vi "CSM-LogViewer.vi"() -> ()   [LabVIEW 2020]
uses:
  Typedef/Def - CSMLog Line - Cluster.ctl
  Typedef/Def - CSMLog Line - File Info - Cluster.ctl
  <userlib>/_NEVSTOP/Communicable State Machine(CSM)/_Support/Priority Queue/Priority Queue.lvclass/Priority Queue.ctl
  5abc820e-fff5-455f-84ac-6161549f095a.vi
  d19c4e55-5bdc-402e-9f7e-e2ad1133e7d6.vi
  <userlib>/_NEVSTOP/Communicable State Machine(CSM)/_Support/Process/CSMP-Async Call.vi
  <userlib>/_NEVSTOP/Communicable State Machine(CSM)/_Support/GlobalEvent/GEvt-Generate Status Log.vi
  <userlib>/_NEVSTOP/Communicable State Machine(CSM)/_Support/Process/CSMP-Broadcast.vi
  <userlib>/_NEVSTOP/Communicable State Machine(CSM)/_Support/GlobalEvent/GEvt-Generate Interrupt Log.vi
  <userlib>/_NEVSTOP/Communicable State Machine(CSM)/_Support/GlobalEvent/GEvt-Generate Register Log.vi
  <userlib>/_NEVSTOP/Communicable State Machine(CSM)/_Support/Process/CSMP-Register Status.vi
  <userlib>/_NEVSTOP/Communicable State Machine(CSM)/_Support/GlobalEvent/GEvt-Generate Unregister Log.vi
  <userlib>/_NEVSTOP/Communicable State Machine(CSM)/_Support/Process/CSMP-Unregister Status.vi
  <userlib>/_NEVSTOP/Communicable State Machine(CSM)/_Support/Process/CSMP-Sync Call.vi
  <userlib>/_NEVSTOP/Communicable State Machine(CSM)/_Support/CSMQ/_CSMObj-Unlock.vi
  <userlib>/_NEVSTOP/Communicable State Machine(CSM)/_Support/Process/CSMP-PostPostMsg.vi
  <userlib>/_NEVSTOP/Communicable State Machine(CSM)/_Support/Process/CSMP-PostSendMsg.vi
  <userlib>/_NEVSTOP/Communicable State Machine(CSM)/_Support/CSMQ/_CSMObj-Lock State.vi
  <userlib>/_NEVSTOP/Communicable State Machine(CSM)/_Support/Common/Splite Reason String Part.vi
  <userlib>/_NEVSTOP/Communicable State Machine(CSM)/_Support/Common/Trim Single line Text.vi
  <userlib>/_NEVSTOP/Communicable State Machine(CSM)/_Support/CSMQ/_CSMOFGV Release.vi
  <userlib>/_NEVSTOP/Communicable State Machine(CSM)/_Support/Common/Remove Comments from Line.vi
  <userlib>/_NEVSTOP/Communicable State Machine(CSM)/_Support/Common/Splite Single-line Message.vi
  <userlib>/_NEVSTOP/Communicable State Machine(CSM)/_Support/Common/Parse Next Single-line State.vi
  <userlib>/_NEVSTOP/Communicable State Machine(CSM)/_Support/CSMQ/_CSMOFGV Dequeue.vi
  <userlib>/_NEVSTOP/Communicable State Machine(CSM)/_Support/CSMQ/_CSMObj-Log Error if in a Remote Session.vi
  <userlib>/_NEVSTOP/Communicable State Machine(CSM)/_Support/GlobalEvent/GEvt-Generate State Change Log.vi
  <userlib>/_NEVSTOP/Communicable State Machine(CSM)/_Support/GlobalEvent/GEvt-Generate Remaining States Log.vi
  <userlib>/_NEVSTOP/Communicable State Machine(CSM)/_Support/GlobalEvent/GEvt-Generate Module Destroyed Log.vi
  <userlib>/_NEVSTOP/Communicable State Machine(CSM)/_Support/GlobalEvent/GEvt-Generate Complete Log.vi
  <userlib>/_NEVSTOP/Communicable State Machine(CSM)/_Support/GlobalEvent/GEvt-Generate Module Created Log.vi
  <userlib>/_NEVSTOP/Communicable State Machine(CSM)/_Support/Common/Format Timestamp.vi
  <userlib>/_NEVSTOP/Communicable State Machine(CSM)/AdvanceAPI/CSM - Revert Arguments-Safe String.vi
  <userlib>/_NEVSTOP/Communicable State Machine(CSM)/AdvanceAPI/CSM - Make String Arguments Safe.vi
  <userlib>/_NEVSTOP/Communicable State Machine(CSM)/AdvanceAPI/CSM - Break Down Multiple States String.vi
  <userlib>/_NEVSTOP/Communicable State Machine(CSM)/AdvanceAPI/CSM - Compact Multiple States.vi
  <userlib>/_NEVSTOP/Communicable State Machine(CSM)/_Support/CSMQ/_Obtain CSM Data Queue.vi
  <userlib>/_NEVSTOP/Communicable State Machine(CSM)/_Support/Priority Queue/Release Priority Queue.vi
  d19c4e55-5bdc-402e-9f7e-e2ad1133e7d6.vi/eb2405bd-5b2e-436b-9bb3-692ecf4a9268.vi
  d19c4e55-5bdc-402e-9f7e-e2ad1133e7d6.vi/c8ad12e3-5e6d-40e1-92e0-1426ef45ec41.vi
  d19c4e55-5bdc-402e-9f7e-e2ad1133e7d6.vi/effcbc1a-e97c-42d4-b61f-d821de102707.vi
  <userlib>/_NEVSTOP/Communicable State Machine(CSM)/_Support/CSMQ/_CSMObj-Message Check.vi
  <userlib>/_NEVSTOP/Communicable State Machine(CSM)/_Support/CSMQ/_CSMObj-Enqueue Cross-Module Message.vi
  <userlib>/_NEVSTOP/Communicable State Machine(CSM)/_Support/CSMQ/_CSMOFGV Get.vi
  <userlib>/_NEVSTOP/Communicable State Machine(CSM)/_Support/FGV-BroadcastRegistry/Cache-Broadcast Registry Search Result.vi
  <userlib>/_NEVSTOP/Communicable State Machine(CSM)/AdvanceAPI/CSM - Register Status Change.vi
  <userlib>/_NEVSTOP/Communicable State Machine(CSM)/AdvanceAPI/CSM - Unregister Status Change.vi
  <userlib>/_NEVSTOP/Communicable State Machine(CSM)/_Support/Common/Hex Str to U8 Data.vi
  <userlib>/_NEVSTOP/Communicable State Machine(CSM)/_Support/Common/Concatenate State with Arguments.vi
  <userlib>/_NEVSTOP/Communicable State Machine(CSM)/_Support/Common/U8 Data to Hex Str.vi
  <userlib>/_NEVSTOP/Communicable State Machine(CSM)/_Support/Priority Queue/Dequeue Element.vi
  <userlib>/_NEVSTOP/Communicable State Machine(CSM)/AdvanceAPI/CSM - Keywords.vi
  <userlib>/_NEVSTOP/Communicable State Machine(CSM)/_Support/Priority Queue/Obtain Priority Queue.vi
  <userlib>/_NEVSTOP/Communicable State Machine(CSM)/_Support/Priority Queue/Enqueue Element.vi
  <userlib>/_NEVSTOP/Communicable State Machine(CSM)/_Support/GlobalEvent/FGV-GlobalEventRef.vi
  <userlib>/_NEVSTOP/Communicable State Machine(CSM)/_Support/CSMQ/_CSMOFGV Obtain.vi
  <userlib>/_NEVSTOP/Communicable State Machine(CSM)/_Support/CSMQ/_CSMOFGV.vi
  <userlib>/_NEVSTOP/Communicable State Machine(CSM)/_Support/Error/CSM Not Allowed Message.vi
  <userlib>/_NEVSTOP/Communicable State Machine(CSM)/_Support/GlobalEvent/FGV-StatusChangeEventRef.vi
  <userlib>/_NEVSTOP/Communicable State Machine(CSM)/_Support/FGV-BroadcastRegistry/global-CSMQ FGV Change Flag.vi
  <userlib>/_NEVSTOP/Communicable State Machine(CSM)/_Support/FGV-BroadcastRegistry/global-Broadcast Cache Change Flag.vi
  <userlib>/_NEVSTOP/Communicable State Machine(CSM)/_Support/BroadcastRegistry/HelperVI/Broadcast Item Key.vi
  <userlib>/_NEVSTOP/Communicable State Machine(CSM)/_Support/FGV-BroadcastRegistry/FGV-BroadcastRegistry.vi
  <userlib>/_NEVSTOP/Communicable State Machine(CSM)/_Support/Message/Parse Register Message.vi
  <userlib>/_NEVSTOP/Communicable State Machine(CSM)/_Support/Message/Parse Unregister Message.vi
  <userlib>/_NEVSTOP/Communicable State Machine(CSM)/addons/API-String-Arugments-Support/_Support/Data To API String Arguments.vi
  <userlib>/_NEVSTOP/Communicable State Machine(CSM)/AdvanceAPI/CSM - Replace Substitution Marks in Messages.vi
  <userlib>/_NEVSTOP/Communicable State Machine(CSM)/_Support/Priority Queue/Priority Queue.lvclass
  <userlib>/_NEVSTOP/Communicable State Machine(CSM)/Communicable State Machine.lvlib
  71ee8597-0d9a-41c2-b129-d09668d4d4ef.vi
  <userlib>/_NEVSTOP/Communicable State Machine(CSM)/addons/API-String-Arugments-Support/API String Arguments Support.lvlib
  <userlib>/_NEVSTOP/Communicable State Machine(CSM)/addons/MassData-Parameter/CSM MassData Parameter Support.lvlib
panel:
  in  "Synchronize":bool
  in  "File Open":bool
  out "State History":string
  in  "Tree":string(tree)
  out "Variant":variant
  out "data":string
  out "offset (in bytes) (0)":i64 format="%.3p"
  out "size (in bytes)":i64 format="%.3p"
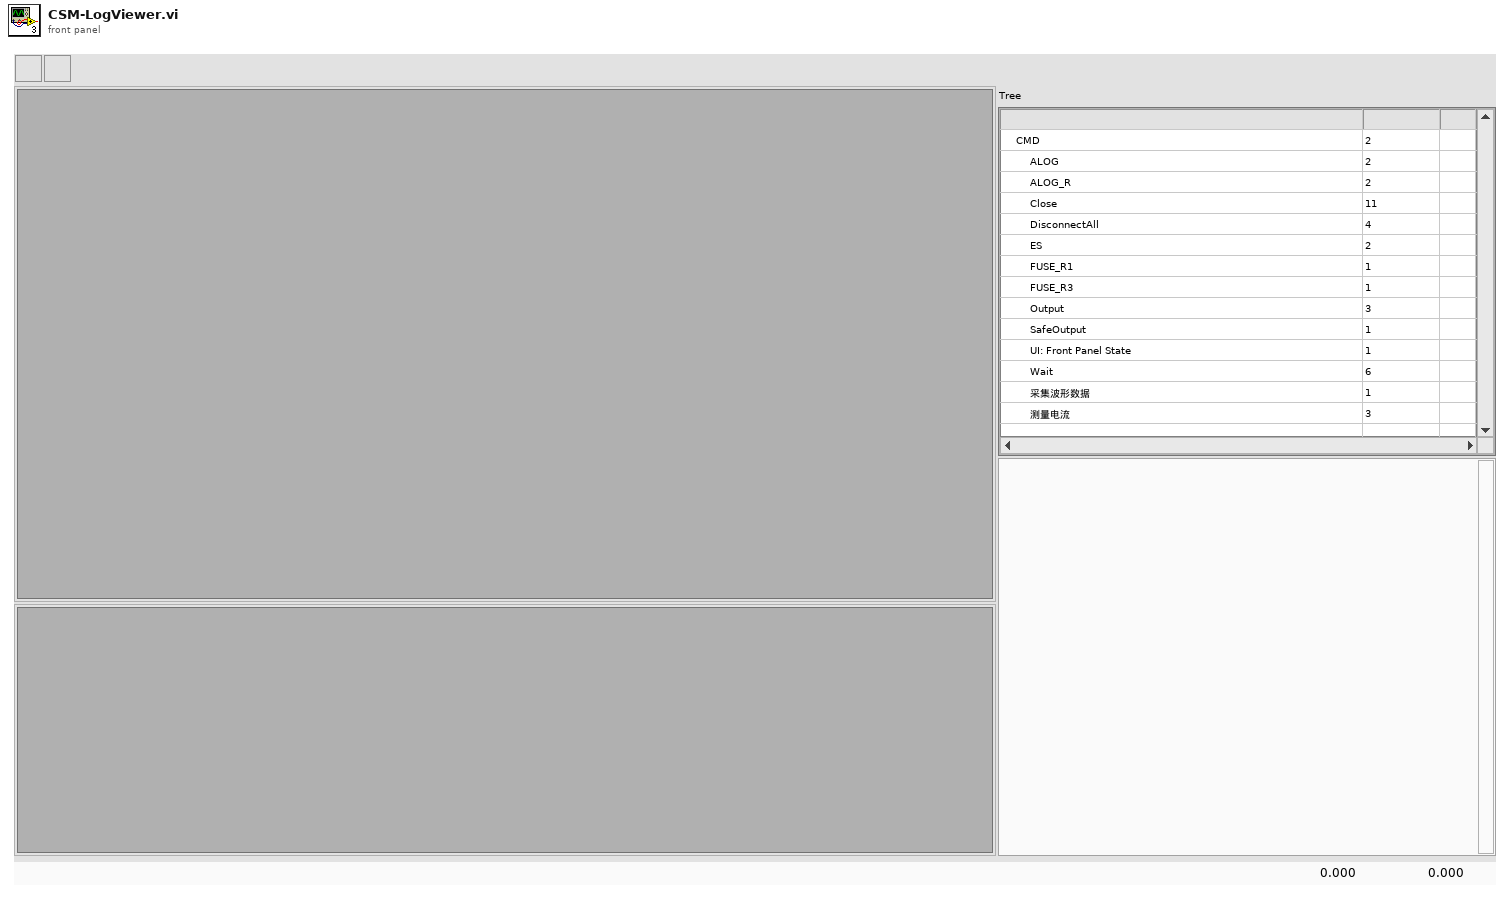
[diagram p1: front panel]
types:
  T1 = typedef "Def - CSMLog Line - Cluster.ctl" = cluster{"Content":string, "FileInfo":T2}
  T2 = typedef "Def - CSMLog Line - File Info - Cluster.ctl" = cluster{"Start":i32, "Length":i32}
  T3 = enum32{"Invalid", "Standard", "Closed", "Hidden", "Minimized", "Maximized"}
  T4 = enum32{"invalid app kind", "Development System", "Run Time System", "Student Edition", "Embedded LabVIEW", "Evaluation", "Custom"}
  T5 = typedef "Communicable State Machine.lvlib/_CSM_Response Source Message.ctl" = cluster{"‘State":string, "’Arguments":string, "’Error":errorcluster}
  T6 = cluster{"Core":cluster{"Current VI Reference":refnum<vi>, "Close Panel on Exit?":bool}, "Your Boolean data":bool, "Your string data":string}
  T7 = cluster{"Current VI Reference":refnum<vi>, "Close Panel on Exit?":bool}
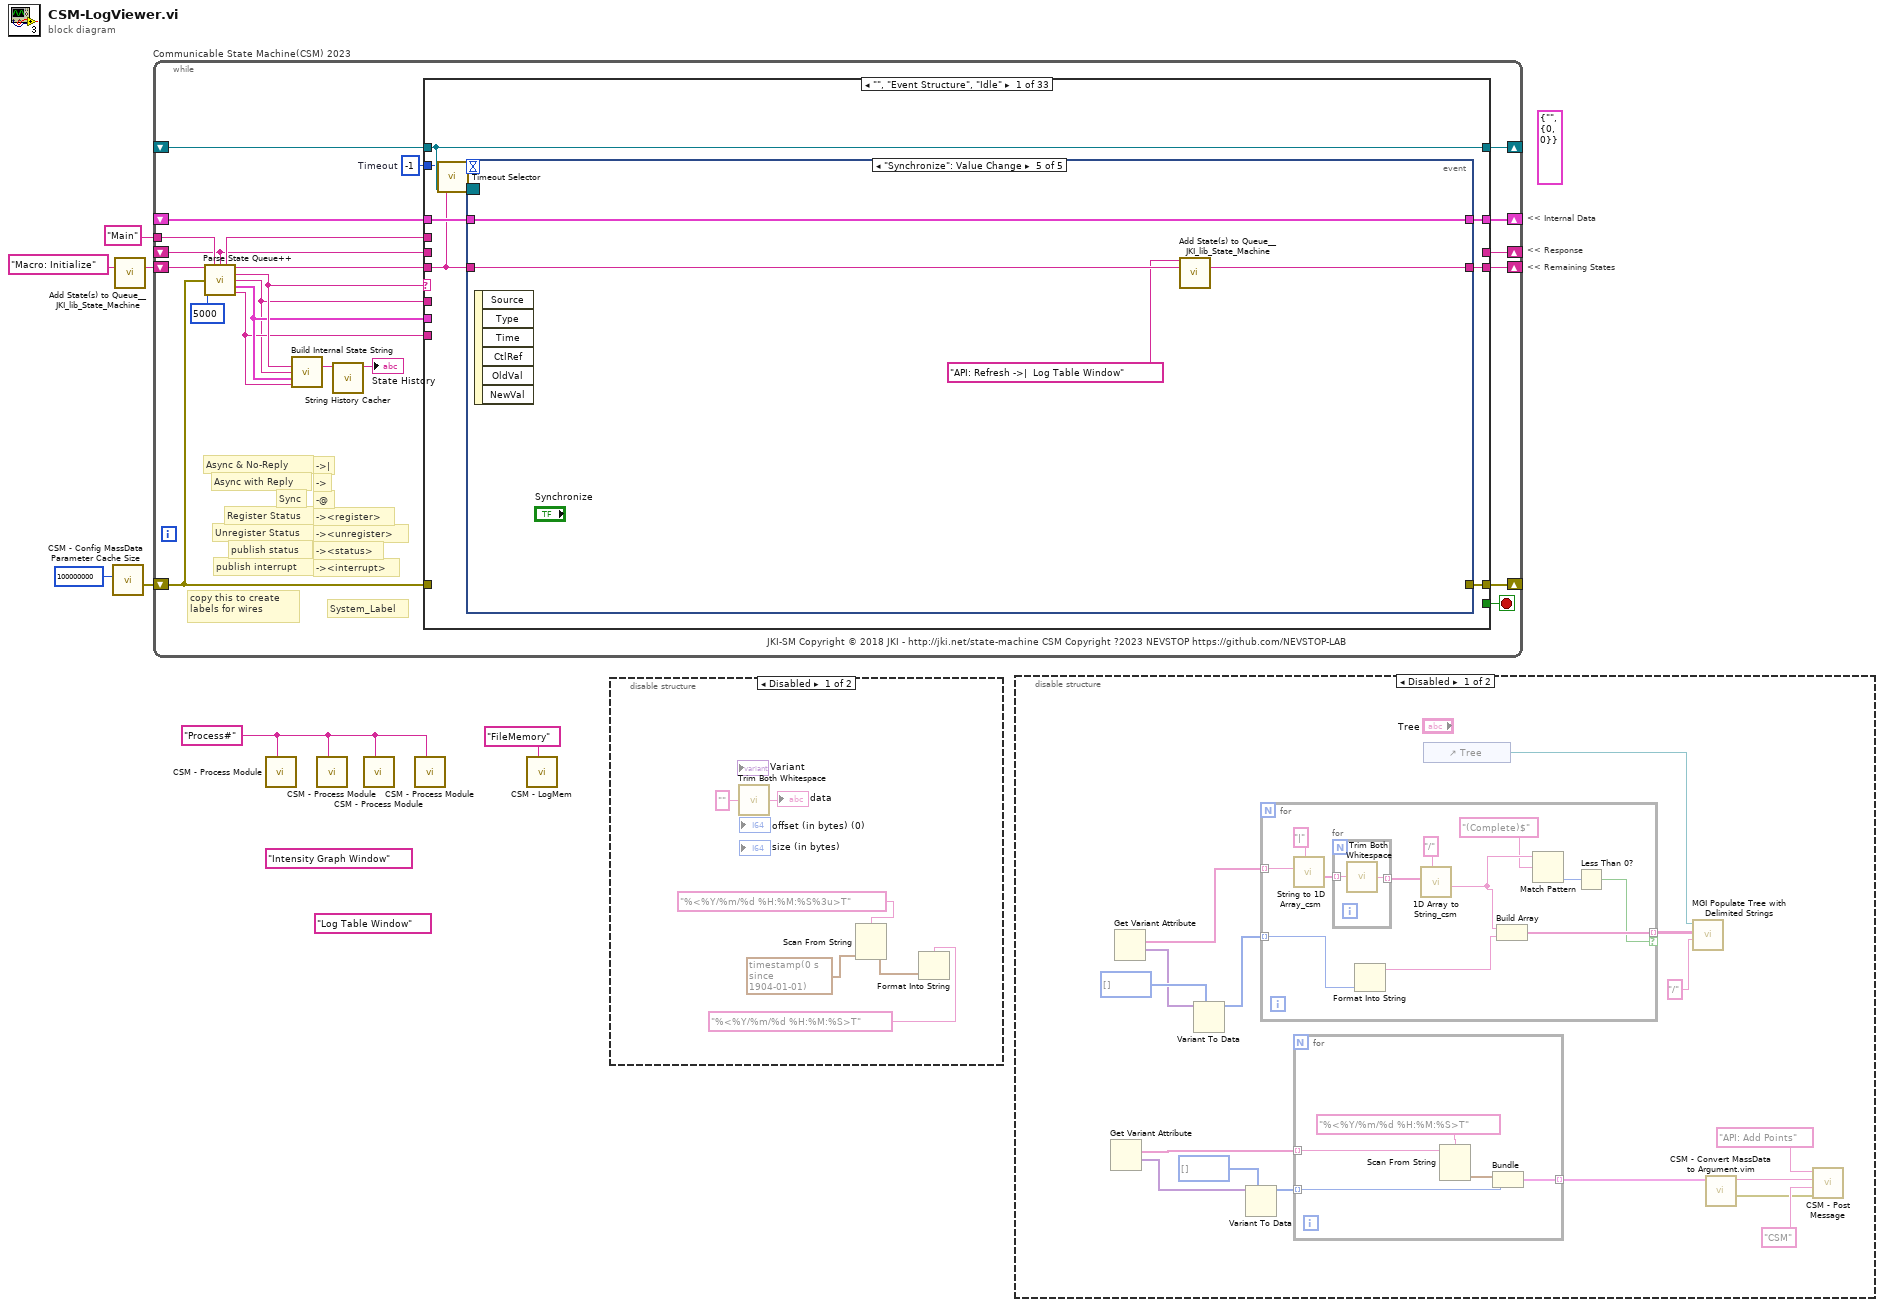
[diagram p0: block diagram]
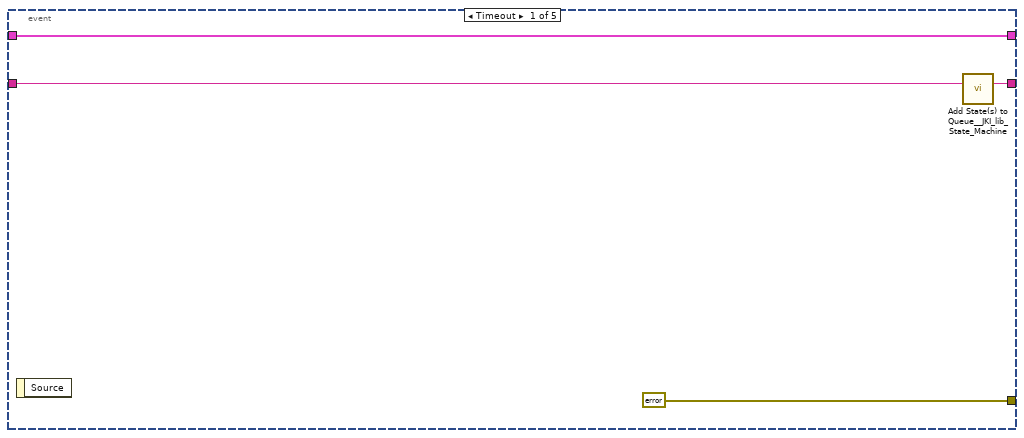
[diagram p4: hidden frame]
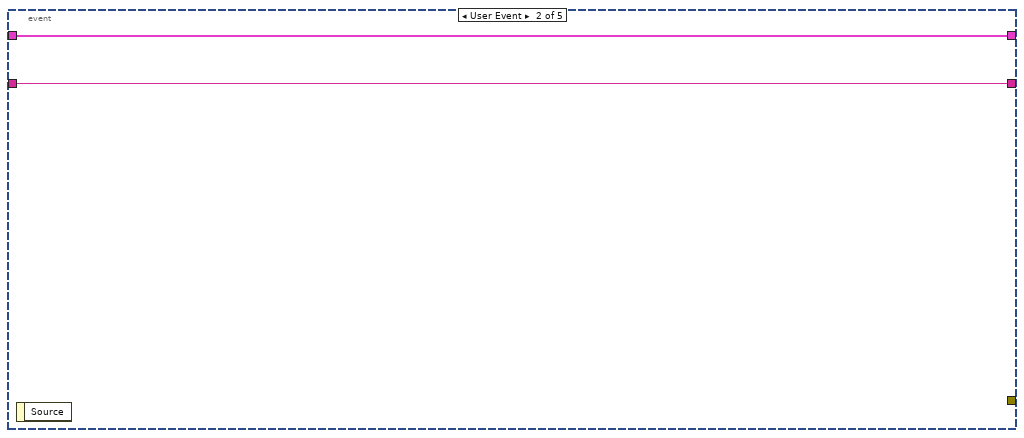
[diagram p5: hidden frame]
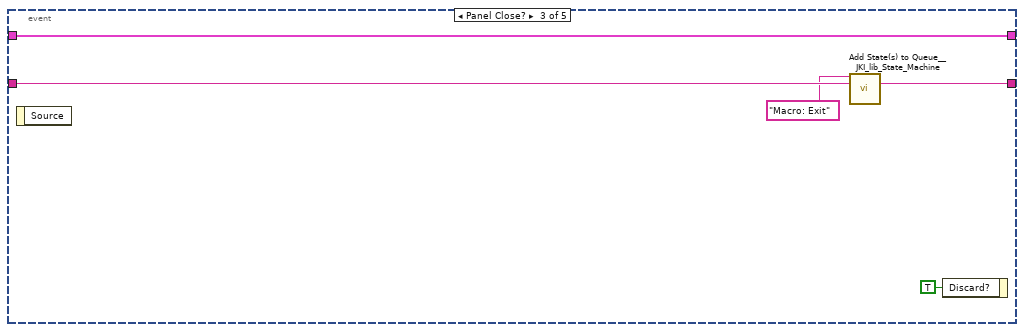
[diagram p6: hidden frame]
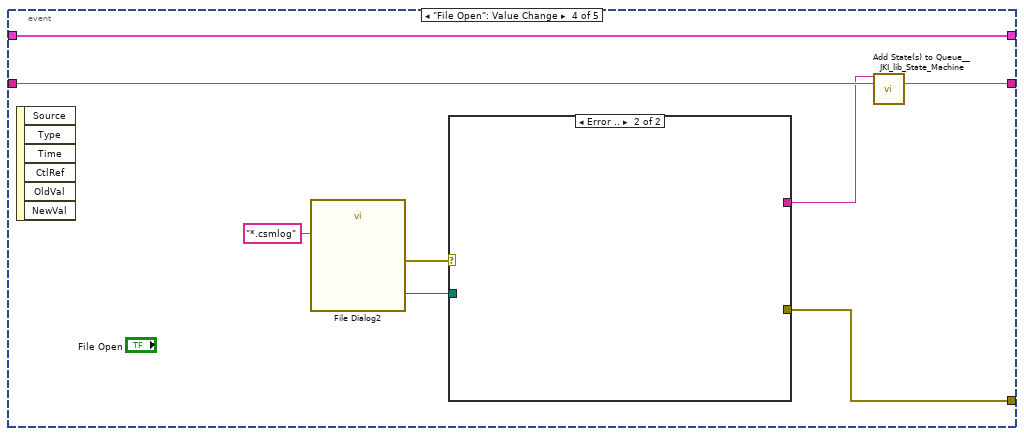
[diagram p7: hidden frame]
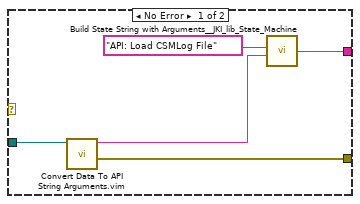
[diagram p8: hidden frame]
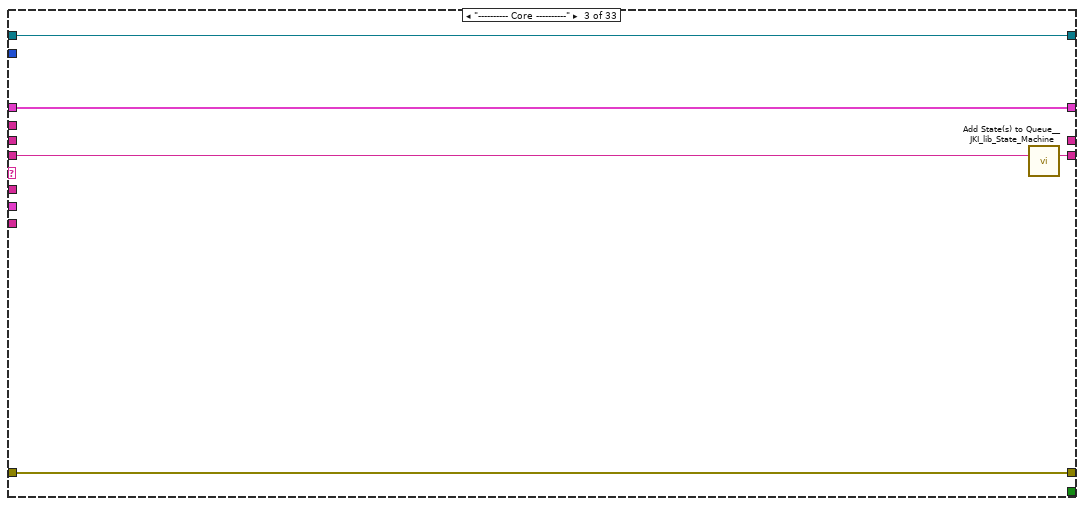
[diagram p10: hidden frame]
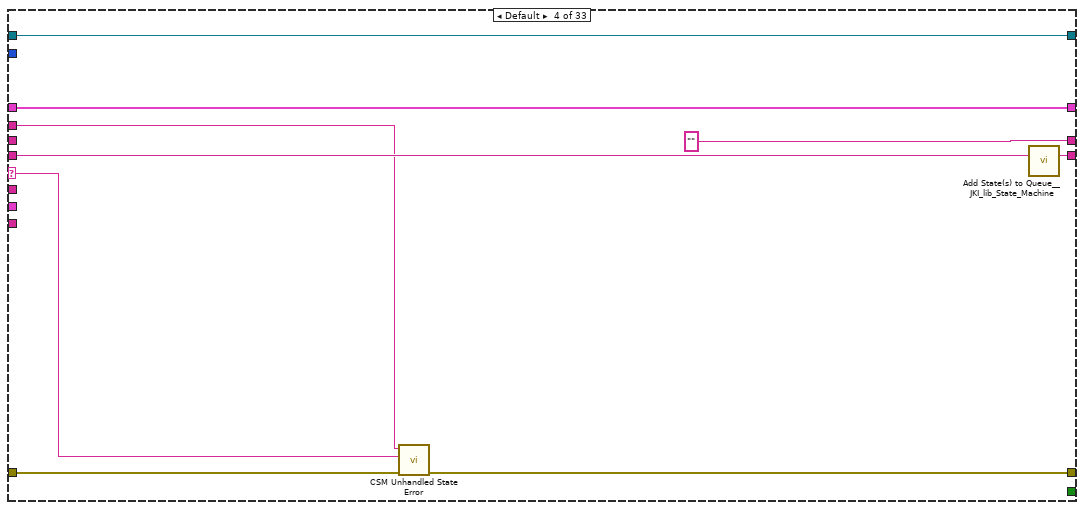
[diagram p11: hidden frame]
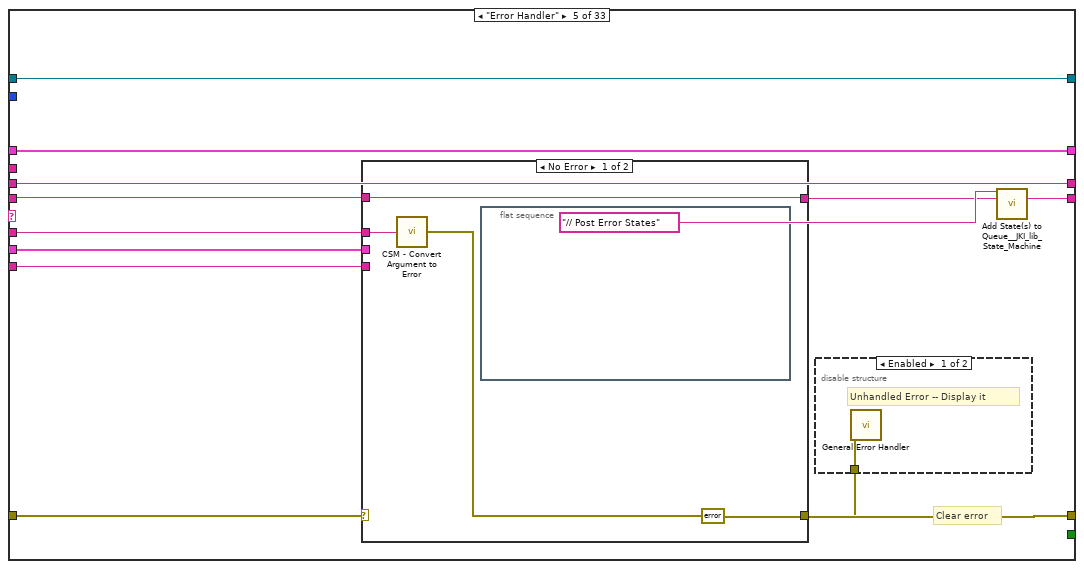
[diagram p12: hidden frame]
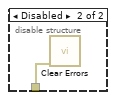
[diagram p13: hidden frame]
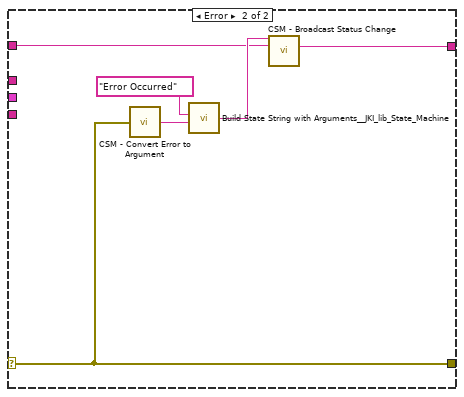
[diagram p14: hidden frame]
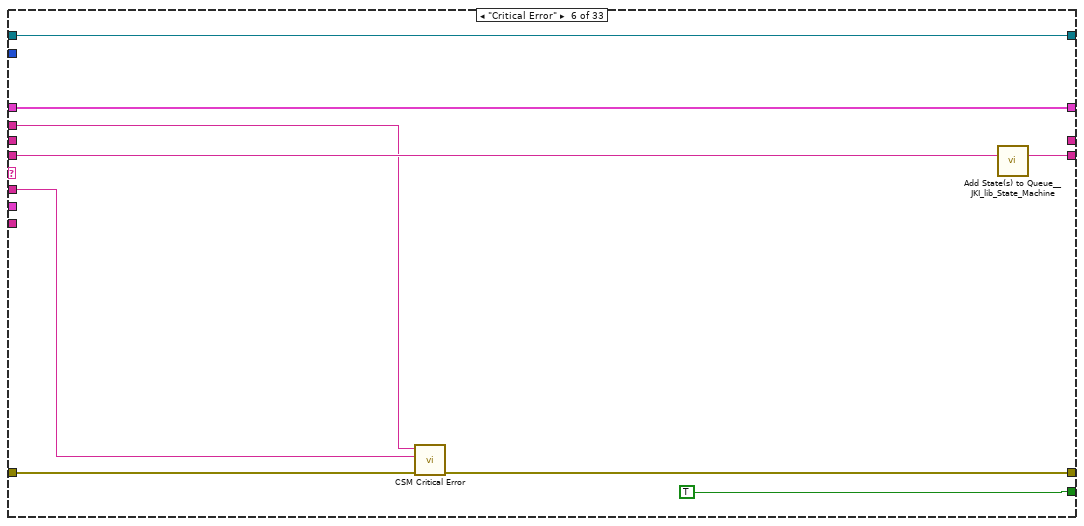
[diagram p15: hidden frame]
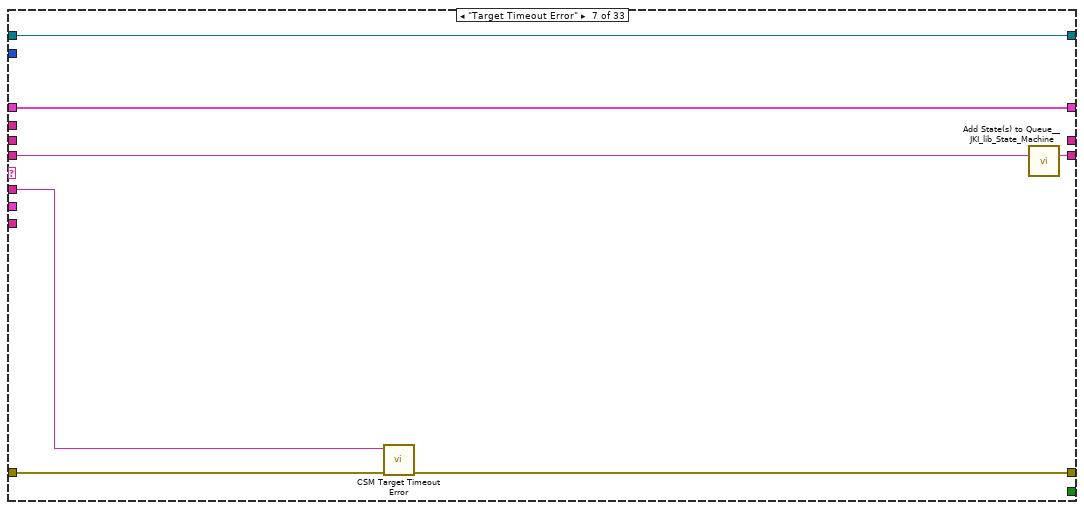
[diagram p16: hidden frame]
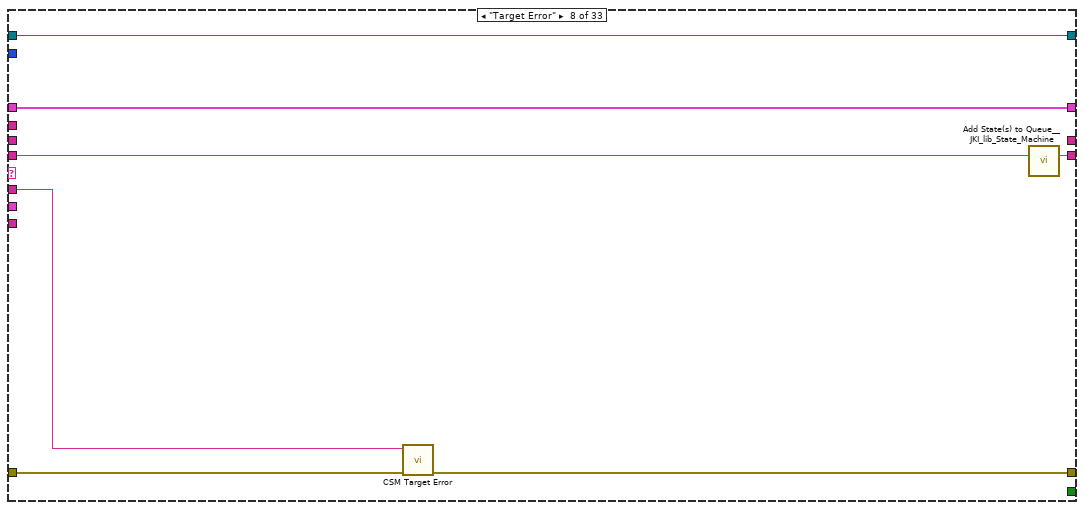
[diagram p17: hidden frame]
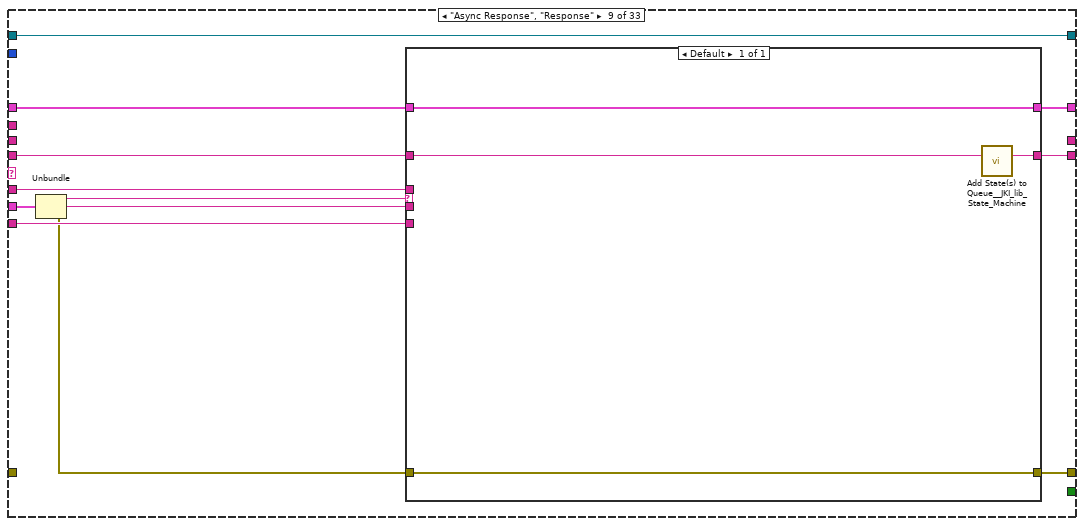
[diagram p18: hidden frame]
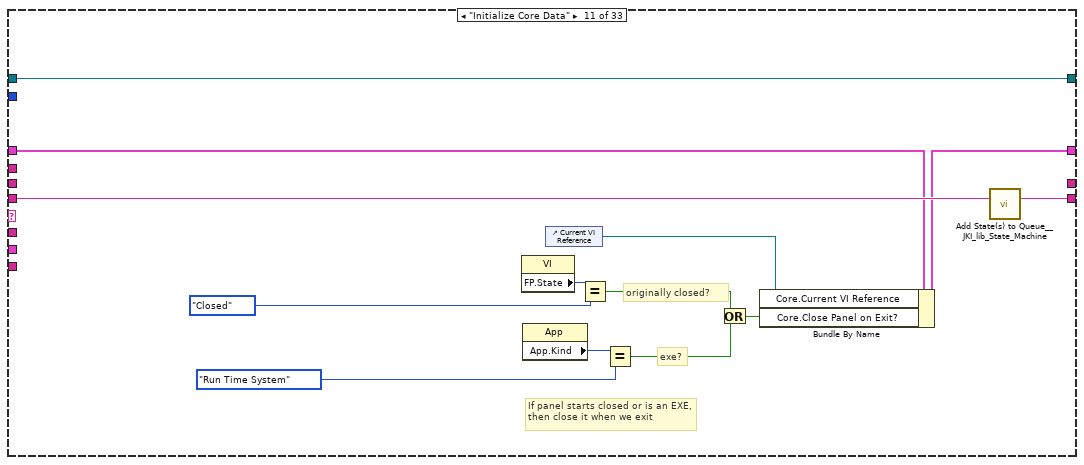
[diagram p20: hidden frame]
diagram:
  (unwired) "Log Table Window" ("CSM Name")
  (unwired) "Intensity Graph Window" ("CSM Name")
  w4 = "Process#" ("Name(\"\" to use uuid)")
  (unwired) T1 {"Content"="", "FileInfo"={"Start"=0, "Length"=0}}
  # "<< Internal Data"
  # "<< Response"
  # "<< Remaining States"
  n1 = call <userlib>:"CSM - Config MassData Parameter Cache Size.vi"("size(1M)"=100000000) -> ("Error out"=w2:errorcluster)  [unwired: 10 in]
  n2 = call <vilib>:"Add State(s) to Queue__JKI_lib_State_Machine.vi"("State(s) in (\"\")"="Macro: Initialize" ("Init State(\"Macro: Initialize\")")) -> ("States Out"=w5:string)  [unwired: 14 in]
  n3 = while "Communicable State Machine(CSM) 2023" {
    shift-right: [w24] -> _
    shift-left: _ -> [w23]
    shift-right: [w27] -> _
    shift-left: w2 -> [w21]
    shift-right: [w26] -> _
    shift-left: w5 -> [w28]
    tunnel: "Main" ("Name(\"\" to use uuid)") -> [w16]
    shift-right: [w19] -> _
    shift-left: _ -> [w9]
    shift-right: [w18] -> _
    shift-left: _ -> [w17]
    stop <- w25 stop-if-true
    w22 = -1  # Timeout
    # "-><interrupt>"
    # "-><status>"
    # "-><unregister>"
    # "-><register>"
    # "-@"
    # "->"
    # "->|"
    # "publish interrupt"
    # "publish status"
    # "Unregister Status"
    # "Register Status"
    # "Sync"
    # "Async with Reply"
    # "Async & No-Reply"
    # "copy this to create labels for wires"
    # "System_Label"
    # "JKI-SM Copyright © 2018 JKI - http://jki.net/state-machine CSM Copyright ?2023 NEVSTOP https://github.com/NEVSTOP-LAB"
    n4 = call <userlib>:"Parse State Queue++.vi"("State Queue"=w28, "Name(\"\" to use uuid)"=w16, "Response Arguments"=w9, "Error In (no error)"=w21, "Response Timeout(5000ms)"=5000 ("Response Timeout(1000ms)")) -> ("Name Used"=w10:string, "Remaining States"=w29:string, "Current State"=w13:string, "Arguments"=w8:string, ">> Response Source Message >>"=w12:T5, ">> Source CSM >>"=w11:string)  [unwired: 5 in]
    n5 = call <userlib>:"Build Internal State String.vi"("State"=w13, "Arguments (\"\")"=w8, ">> Response Source Message >>"=w12, "Source (\"\")"=w11) -> ("State with Arguments"=w14:string)  [unwired: 11 in]
    n6 = call <userlib>:"String History Cacher.vi"("String"=w14) -> ("String Cache"=→"State History":string)  [unwired: 10 in]
    n7 = case shown="\"\", \"Event Structure\", \"Idle\"" w13 {
      selector: w13 -> [_ _ _ w76 _ _ _ _ _ _ _ _ _ _ _ _ _ _ _ _ _ _ _ _ _ _ _ _ _ _ _ _ _]
      tunnel: w29 -> [w30 w68 w73 w82 w88 w114 w122 w129 w139 w148 w161 w166 w170 w177 w183 w187 w194 w198 w202 w206 w212 w224 w297 w334 w362 w367 w381 w384 w399 w405 w409 w413 w417]
      tunnel: w8 -> [_ _ _ _ w86 w110 w117 w125 w133 _ _ _ _ _ _ _ _ _ _ _ w208 w219 _ _ _ _ _ _ w387 _ _ _ _]
      tunnel: w23 -> [w36 w67 w70 w80 w94 w115 w120 w127 w137 w147 w155 w164 w168 _ w179 w185 w193 w197 w200 w204 w210 w221 w296 w333 w360 w365 w379 w383 w402 w404 w407 w411 w415]
      tunnel: [w35 _ w71 w74 errorcluster {"status"=FALSE, "code"=0, "source"=""} ("error out") w107 w116 w123 w136 _ _ _ _ _ w180 _ w188 w196 _ _ w209 w222 w290 w328 _ _ _ _ w385 _ _ _ _] -> w27
      tunnel: w21 -> [_ _ w71 w75 w92 w108 w118 w124 _ _ _ _ _ _ _ _ _ _ _ _ _ _ _ _ _ _ _ _ _ _ _ _ _]
      tunnel: [w37 w68 w72 w81 w90 w113 w121 w128 w140 w148 w160 w165 w169 w176 w182 w186 w194 w198 w201 w205 w211 w223 w297 w334 w361 w366 w380 w384 w400 w405 w408 w412 w416] -> w26
      tunnel: [_ _ _ _ _ TRUE _ _ _ _ _ TRUE _ _ _ _ _ _ _ _ _ _ _ _ _ _ _ _ _ _ _ _ _] -> w25
      tunnel: [w34 w67 w70 w80 w94 w115 w120 w127 w138 w147 w159 w164 w168 w175 w179 w185 w193 w197 w200 w204 w210 w221 w296 w333 w360 w365 w379 w383 w402 w404 w407 w411 w415] -> w24
      tunnel: w22 -> [w32 _ _ _ _ _ _ _ _ _ _ _ _ _ _ _ _ _ _ _ _ _ _ _ _ _ _ _ _ _ _ _ _]
      tunnel: w11 -> [_ _ _ _ w85 _ _ _ w134 _ _ _ _ _ _ _ _ _ _ _ _ _ _ _ _ _ _ _ _ _ _ _ _]
      tunnel: w12 -> [_ _ _ _ w84 _ _ _ w135 _ _ _ _ _ _ _ _ _ _ _ _ _ _ _ _ _ _ _ _ _ _ _ _]
      tunnel: [_ _ _ "" w83 _ _ _ _ _ _ _ _ _ _ _ _ _ _ _ _ _ _ _ _ _ _ _ _ _ _ _ _] -> w19
      tunnel: [w33 w66 w69 w78 w93 w111 w119 w126 w141 w146 w149 w162 w167 w171 w178 w184 w192 w195 w199 w203 w207 w218 w295 w332 w359 w363 w372 w382 w401 w403 w406 w410 w414] -> w18
      tunnel: w17 -> [w33 w66 w69 w78 w93 w111 w119 w126 w141 w146 w149 w162 w167 w171 w178 w184 _ w195 w199 w203 w207 w218 w295 w332 w359 w363 w372 w382 w401 w403 w406 w410 w414]
      tunnel: w10 -> [_ _ _ w77 _ w109 _ _ _ _ _ _ _ _ _ _ w191 _ _ _ _ _ _ _ _ _ w370 _ _ _ _ _ _]
      tunnel: w9 -> [_ _ _ _ w83 _ _ _ _ _ _ _ _ _ _ _ _ _ _ _ _ _ _ _ _ _ _ _ _ _ _ _ _]
      frame "", "Event Structure", "Idle" {
        n8 = call <userlib>:"Timeout Selector.vi"("Remaining States"=w30, "Timeout Expected"=w32) -> ("Timeout"=w31:i32)  [unwired: 5 in]
        n9 = event shown="[4] \"Synchronize\": Value Change" {
          selector: w33 -> [_ _ _ _ _]
          dyn-events: _ -> [_ _ _ _ _]
          timeout: w31 -> [_ _ _ _ _]
          tunnel: w30 -> [w41 w42 w48 w54 w63]
          tunnel: [w40 w42 w47 w55 w64] -> w37
          tunnel: w36 -> [w39 w43 w46 w56 w65]
          tunnel: [errorcluster {"status"=FALSE, "code"=0, "source"=""} ("error out") _ _ w51 _] -> w35
          tunnel: [w39 w43 w46 w56 w65] -> w34
          event Timeout {
            n10 = event-data() -> ()  [unwired: 1 in, 1 out]
            n11 = call <vilib>:"Add State(s) to Queue__JKI_lib_State_Machine.vi"("State(s) in (\"\")"=w41) -> ("States Out"=w40:string)  [unwired: 14 in]
          }
          event User Event {
            n12 = event-data() -> ()  [unwired: 1 in, 1 out]
          }
          event Panel Close? {
            n13 = event-data() -> ()  [unwired: 1 in, 1 out]
            n14 = call <vilib>:"Add State(s) to Queue__JKI_lib_State_Machine.vi"("State(s) in Front (\"\")"="Macro: Exit", "State(s) in (\"\")"=w48) -> ("States Out"=w47:string)  [unwired: 13 in]
            n15 = event-data("Discard?"=TRUE) -> ()  [unwired: 1 in, 1 out]
          }
          event "File Open": Value Change {
            n16 = event-data() -> ()  [unwired: 1 in, 6 out]
            n17 = call "File Dialog2"("pattern (all files)"="*.csmlog") -> ("selected path"=w52:path, "error out"=w50:errorcluster)  [unwired: 11 in, 2 out]
            n18 = case shown="Error .." w50 {
              tunnel: [w61 _] -> w53
              tunnel: w52 -> [w59 _]
              tunnel: [w57 _] -> w51
              frame No Error {
                n19 = call "Convert Data To API String Arguments.vim"("data"=w59) -> ("error out"=w57:errorcluster, "String"=w58:string)  [unwired: 7 in]
                n20 = call <vilib>:"Build State String with Arguments__JKI_lib_State_Machine.vi"("Arguments (\"\")"=w58, "State"="API: Load CSMLog File" ("State(s) in Front (\"\")")) -> ("State with Arguments"=w61:string)  [unwired: 4 in]
              }
              frame Error {
              }
            }
            n21 = call <vilib>:"Add State(s) to Queue__JKI_lib_State_Machine.vi"("State(s) in Front (\"\")"=w53, "State(s) in (\"\")"=w54) -> ("States Out"=w55:string)  [unwired: 13 in]
          }
          event "Synchronize": Value Change {
            n22 = event-data() -> ()  [unwired: 1 in, 6 out]
            n23 = call <vilib>:"Add State(s) to Queue__JKI_lib_State_Machine.vi"("State(s) in Front (\"\")"="API: Refresh ->|  Log Table Window" ("State(s) in Front (\"\")"), "State(s) in (\"\")"=w63) -> ("States Out"=w64:string)  [unwired: 13 in]
          }
        }
      }
      frame "CSM Documentation" {
      }
      frame "---------- Core ----------" {
        n24 = call <vilib>:"Add State(s) to Queue__JKI_lib_State_Machine.vi"("State(s) in (\"\")"=w73) -> ("States Out"=w72:string)  [unwired: 14 in]
      }
      frame Default {
        n25 = call <userlib>:"CSM Unhandled State Error.vi"("error in (no error)"=w75, "State"=w76, "CSM"=w77) -> ("error out"=w74:errorcluster)  [unwired: 8 in]
        n26 = call <vilib>:"Add State(s) to Queue__JKI_lib_State_Machine.vi"("State(s) in (\"\")"=w82) -> ("States Out"=w81:string)  [unwired: 14 in]
      }
      frame "Error Handler" {
        # "Clear error"
        n27 = case shown="No Error" w92 {
          selector: w92 -> [_ w101]
          tunnel: [w99 w103] -> w89
          tunnel: w88 -> [w99 w102]
          tunnel: [w98 w101] -> w87
          tunnel: w86 -> [w100 _]
          tunnel: w85 -> [_ _]
          tunnel: w84 -> [_ _]
          frame No Error {
            n28 = call <userlib>:"CSM - Convert Argument to Error.vi"("Argument"=w100) -> ("error"=w98:errorcluster)  [unwired: 4 in]
            n29 = flat-sequence {
              frame #0 {
              }
            }
          }
          frame Error {
            n30 = call <userlib>:"CSM - Convert Error to Argument.vi"("error in (no error)"=w101) -> ("Arguments"=w105:string)  [unwired: 4 in]
            n31 = call <vilib>:"Build State String with Arguments__JKI_lib_State_Machine.vi"("Arguments (\"\")"=w105, "State"="Error Occurred" ("Status with Arguments")) -> ("State with Arguments"=w104:string)  [unwired: 4 in]
            n32 = call <userlib>:"CSM - Broadcast Status Change.vi"("Status with Arguments"=w104, "State Queue"=w102) -> ("Remaining States"=w103:string)  [unwired: 13 in]
          }
        }
        n33 = disable-structure shown="Enabled" {
          disable-tunnel: w87 -> [w96 w97]
          frame Enabled {
            # "Unhandled Error -- Display it"
            n34 = call <vilib>:"General Error Handler.vi"("error in (no error)"=w96) -> ()  [unwired: 10 in, 5 out]
          }
          frame Disabled {
            n35 = call <vilib>:"Clear Errors.vi"("error in (no error)"=w97) -> ()  [unwired: 5 in, 2 out]
          }
        }
        n36 = call <vilib>:"Add State(s) to Queue__JKI_lib_State_Machine.vi"("State(s) in Front (\"\")"="// Post Error States", "State(s) in (\"\")"=w89) -> ("States Out"=w90:string)  [unwired: 13 in]
      }
      frame "Critical Error" {
        n37 = call <userlib>:"CSM Critical Error.vi"("error in (no error)"=w108, "input"=w110, "CSM Name"=w109) -> ("error out"=w107:errorcluster)  [unwired: 8 in]
        n38 = call <vilib>:"Add State(s) to Queue__JKI_lib_State_Machine.vi"("State(s) in (\"\")"=w114) -> ("States Out"=w113:string)  [unwired: 14 in]
      }
      frame "Target Timeout Error" {
        n39 = call <userlib>:"CSM Target Timeout Error.vi"("error in (no error)"=w118, "CSM Name"=w117) -> ("error out"=w116:errorcluster)  [unwired: 9 in]
        n40 = call <vilib>:"Add State(s) to Queue__JKI_lib_State_Machine.vi"("State(s) in (\"\")"=w122) -> ("States Out"=w121:string)  [unwired: 14 in]
      }
      frame "Target Error" {
        n41 = call <userlib>:"CSM Target Error.vi"("error in (no error)"=w124, "CSM Name"=w125) -> ("error out"=w123:errorcluster)  [unwired: 9 in]
        n42 = call <vilib>:"Add State(s) to Queue__JKI_lib_State_Machine.vi"("State(s) in (\"\")"=w129) -> ("States Out"=w128:string)  [unwired: 14 in]
      }
      frame "Async Response", "Response" {
        n43 = Unbundle(w135) -> ("‘State"=w132:string, "’Arguments"=w131:string, "’Error"=w130:errorcluster)
        n44 = case shown="Default" w132 {
          tunnel: [w142] -> w140
          tunnel: w139 -> [w143]
          tunnel: [w145] -> w138
          tunnel: w137 -> [w145]
          tunnel: [w144] -> w136
          tunnel: w130 -> [w144]
          tunnel: w134 -> [_]
          tunnel: w133 -> [_]
          tunnel: w131 -> [_]
          frame Default {
            n45 = call <vilib>:"Add State(s) to Queue__JKI_lib_State_Machine.vi"("State(s) in (\"\")"=w143) -> ("States Out"=w142:string)  [unwired: 14 in]
          }
        }
      }
      frame "Async Message Posted" {
      }
      frame "Initialize Core Data" {
        # "originally closed?"
        # "exe?"
        # "If panel starts closed or is an EXE, then close it when we exit"
        n46 = property class="VI"() -> ("FP.State"=w152:T3)  [unwired: 2 in, 2 out]
        n47 = property class="App"() -> ("App.Kind"=w158:T4)  [unwired: 2 in, 2 out]
        n48 = control-ref of="Current VI Reference"() -> (w153:refnum<vi>)
        n49 = Equal?(x=w152, y=T3."Closed" ("Front Panel Window:State")) -> (x = y?=w150:bool)
        n50 = Equal?(x=w158, y=T4."Run Time System" ("Application:Kind")) -> (x = y?=w156:bool)
        n51 = Or(x=w150, y=w156) -> (x .or. y?=w154:bool)
        n52 = Bundle By Name(cluster=w155, "Core.Current VI Reference"=w153, "Core.Close Panel on Exit?"=w154) -> (w159:T6)
        n53 = call <vilib>:"Add State(s) to Queue__JKI_lib_State_Machine.vi"("State(s) in (\"\")"=w161) -> ("States Out"=w160:string)  [unwired: 14 in]
      }
      frame "Exit" {
        n54 = call <vilib>:"Add State(s) to Queue__JKI_lib_State_Machine.vi"("State(s) in (\"\")"=w166) -> ("States Out"=w165:string)  [unwired: 14 in]
      }
      frame "---------- Data ----------" {
        n55 = call <vilib>:"Add State(s) to Queue__JKI_lib_State_Machine.vi"("State(s) in (\"\")"=w170) -> ("States Out"=w169:string)  [unwired: 14 in]
      }
      frame "Data: Initialize" {
        w172 = T7 {"Current VI Reference"=refnum, "Close Panel on Exit?"=FALSE}  # Core
        w174 = TRUE  # Your Boolean data
        w173 = ""  # Your string data
        n56 = Bundle("Core"=w172, "Your Boolean data"=w174, "Your string data"=w173) -> (w175:T6)  [unwired: 1 in]
        n57 = call <vilib>:"Add State(s) to Queue__JKI_lib_State_Machine.vi"("State(s) in (\"\")"=w177) -> ("States Out"=w176:string)  [unwired: 14 in]
      }
      frame "Data: Cleanup" {
        n58 = Unbundle By Name(w179) -> ("Core.Current VI Reference"=w181:refnum<vi>)
        n59 = Close Reference(reference=w181) -> (error out=w180:errorcluster)  [unwired: 1 in]
        n60 = call <vilib>:"Add State(s) to Queue__JKI_lib_State_Machine.vi"("State(s) in (\"\")"=w183) -> ("States Out"=w182:string)  [unwired: 14 in]
      }
      frame "---------- Events ----------" {
        n61 = call <vilib>:"Add State(s) to Queue__JKI_lib_State_Machine.vi"("State(s) in (\"\")"=w187) -> ("States Out"=w186:string)  [unwired: 14 in]
      }
      frame "Events: Register" {
        n62 = call <userlib>:"CSM - Get New State Notifier Event.vi"("Name(\"\" to use uuid) in"=w191) -> ("Error out"=w189:errorcluster, "New State Notifier Event"=w190:refnum<user-event>)  [unwired: 9 in]
        n63 = register-events(error in=w189, w190) -> (reference out=w192:refnum<event-registration>, error out=w188:errorcluster)  [unwired: 1 in]
      }
      frame "Events: Unregister" {
        n64 = Unregister For Events(event registration refnum=w195) -> (error out=w196:errorcluster)  [unwired: 1 in]
      }
      frame "---------- UI ----------" {
        n65 = call <vilib>:"Add State(s) to Queue__JKI_lib_State_Machine.vi"("State(s) in (\"\")"=w202) -> ("States Out"=w201:string)  [unwired: 14 in]
      }
      frame "UI: Initialize" {
        n66 = call <vilib>:"Add State(s) to Queue__JKI_lib_State_Machine.vi"("State(s) in (\"\")"=w206) -> ("States Out"=w205:string)  [unwired: 14 in]
      }
      frame "UI: Cursor Set" {
        # "Argument"
        n67 = disable-structure shown="Default" {
          disable-tunnel: [w214 w217] -> w209
          disable-tunnel: w208 -> [w213 _]
          frame condition #0 (active) {
            n68 = case shown="\"Idle\", Default" w213 {
              tunnel: [w215 w216] -> w214
              frame "Idle", Default {
                n69 = call <vilib>:"Unset Busy.vi"() -> ("error out"=w215:errorcluster)  [unwired: 11 in]
              }
              frame "Busy" {
                n70 = call <vilib>:"Set Busy.vi"() -> ("error out"=w216:errorcluster)  [unwired: 10 in, 1 out]
              }
            }
          }
          frame condition #1 {
          }
        }
        n71 = call <vilib>:"Add State(s) to Queue__JKI_lib_State_Machine.vi"("State(s) in (\"\")"=w212) -> ("States Out"=w211:string)  [unwired: 14 in]
      }
      frame "UI: Front Panel State" {
        # "Argument"
        n72 = Unbundle By Name(w221) -> ("Core.Current VI Reference"=w220:refnum<vi>)
        n73 = case shown="\"Minimize\", \"Minimized\"" w219 {
          tunnel: [w231 w244 w255 w267 w279] -> w222
          tunnel: w220 -> [w230 w242 w254 w266 w278]
          frame "Open", "Standard", Default {
            w225 = T3."Standard" ("State")
            n74 = property class="VI"(reference=w230) -> (reference out=w228:refnum<vi>, error out=w229:errorcluster, "FP.State"=w227:T3)  [unwired: 1 in]
            n75 = Not Equal?(x=w227, y=w225) -> (x != y?=w226:bool)
            n76 = case shown="True" w226 {
              tunnel: [w235 w237] -> w231
              tunnel: w229 -> [w234 w237]
              tunnel: w228 -> [w233 _]
              tunnel: w225 -> [w232 _]
              frame True {
                n77 = invoke class="VI" method="FP.Open"(reference=w233, error in=w234, "Activate"=TRUE, "State"=w232) -> (error out=w235:errorcluster)  [unwired: 1 in, 4 out]
              }
              frame False {
              }
            }
          }
          frame "Close", "Closed" {
            n78 = property class="VI"(reference=w242) -> (reference out=w241:refnum<vi>, error out=w243:errorcluster, "FP.State"=w239:T3)  [unwired: 1 in]
            n79 = Not Equal?(x=w239, y=T3."Closed" ("Front Panel Window:State")) -> (x != y?=w238:bool)
            n80 = case shown="True" w238 {
              tunnel: [w245 w248] -> w244
              tunnel: w243 -> [w245 w247]
              tunnel: w241 -> [_ w246]
              frame False {
              }
              frame True {
                n81 = invoke class="VI" method="FP.Close"(reference=w246, error in=w247) -> (error out=w248:errorcluster)  [unwired: 1 in, 2 out]
              }
            }
          }
          frame "Hidden", "Hide" {
            w249 = T3."Hidden" ("State")
            n82 = property class="VI"(reference=w254) -> (reference out=w252:refnum<vi>, error out=w253:errorcluster, "FP.State"=w251:T3)  [unwired: 1 in]
            n83 = Not Equal?(x=w251, y=w249) -> (x != y?=w250:bool)
            n84 = case shown="True" w250 {
              tunnel: [w259 w260] -> w255
              tunnel: w253 -> [w258 w260]
              tunnel: w252 -> [w257 _]
              tunnel: w249 -> [w256 _]
              frame True {
                n85 = invoke class="VI" method="FP.Open"(reference=w257, error in=w258, "State"=w256) -> (error out=w259:errorcluster)  [unwired: 2 in, 4 out]
              }
              frame False {
              }
            }
          }
          frame "Minimize", "Minimized" {
            w261 = T3."Minimized" ("State")
            n86 = property class="VI"(reference=w266) -> (reference out=w264:refnum<vi>, error out=w265:errorcluster, "FP.State"=w263:T3)  [unwired: 1 in]
            n87 = Not Equal?(x=w263, y=w261) -> (x != y?=w262:bool)
            n88 = case shown="False" w262 {
              tunnel: [w271 w272] -> w267
              tunnel: w265 -> [w270 w272]
              tunnel: w264 -> [w269 _]
              tunnel: w261 -> [w268 _]
              frame True {
                n89 = invoke class="VI" method="FP.Open"(reference=w269, error in=w270, "State"=w268) -> (error out=w271:errorcluster)  [unwired: 2 in, 4 out]
              }
              frame False {
              }
            }
          }
          frame "Maximize", "Maximized" {
            w273 = T3."Maximized" ("State")
            n90 = property class="VI"(reference=w278) -> (reference out=w276:refnum<vi>, error out=w277:errorcluster, "FP.State"=w275:T3)  [unwired: 1 in]
            n91 = Not Equal?(x=w275, y=w273) -> (x != y?=w274:bool)
            n92 = case shown="True" w274 {
              tunnel: [w283 w284] -> w279
              tunnel: w277 -> [w282 w284]
              tunnel: w276 -> [w281 _]
              tunnel: w273 -> [w280 _]
              frame True {
                n93 = invoke class="VI" method="FP.Open"(reference=w281, error in=w282, "State"=w280) -> (error out=w283:errorcluster)  [unwired: 2 in, 4 out]
              }
              frame False {
              }
            }
          }
        }
        n94 = call <vilib>:"Add State(s) to Queue__JKI_lib_State_Machine.vi"("State(s) in (\"\")"=w224) -> ("States Out"=w223:string)  [unwired: 14 in]
      }
      frame "UI: Insert Intensity Graph Window" {
        n95 = call <userlib>:"CSM - Check If Module Exists.vi"("CSM Name"="Intensity Graph Window") -> ("Error out"=w287:errorcluster, "Exist?"=w289:bool, "CSM Name(dup)"=w286:string)  [unwired: 8 in]
        n96 = case shown="False" w289 {
          tunnel: [w303 w321] -> w288
          tunnel: w287 -> [w304 w321]
          tunnel: w286 -> [w302 w320]
          tunnel: [w302 w320] -> w285
          frame False {
            n97 = vi-ref "CSM Intensity Graph Window.vi"() -> (w305:refnum<vi>)
            n98 = property class="VI (strict)"(reference=w305, error in=w304) -> (reference out=w308:refnum<vi>, error out=w307:errorcluster, "Path"=w306:path)
            n99 = Open VI Reference(type specifier VI Refnum (for type only)=w308, vi path=w306, options=128, error in (no error)=w307) -> (vi reference=w300:refnum<vi>, error out=w301:errorcluster)  [unwired: 2 in]
            n100 = disable-structure shown="Enabled" {
              disable-tunnel: w301 -> [w317 w319]
              disable-tunnel: w300 -> [w316 w318]
              disable-tunnel: [w315 w318] -> w299
              disable-tunnel: [w313 w319] -> w298
              frame Disabled {
                n101 = invoke class="VI (strict)" method="FP.Open"(reference=w316, error in=w317, "State"=T3."Hidden") -> (reference out=w315:refnum<vi>, error out=w314:errorcluster)  [unwired: 2 in, 3 out]
                n102 = call <userlib>:"MGI Clear Error.vi"("Error In"=w314) -> ("Error Out"=w313:errorcluster)  [unwired: 6 in]
              }
              frame Enabled {
              }
            }
            n103 = call-by-ref "Start Asynchronous Call"(reference=w299, error in=w298, "Name(\"\" to use uuid)"=w302) -> (reference out=w310:refnum<vi>, error out=w309:errorcluster)  [unwired: 11 in]
            n104 = Close Reference(reference=w310, error in (no error)=w309) -> (error out=w303:errorcluster)
          }
          frame True {
          }
        }
        n105 = call <userlib>:"CSM - Query CSM VI Ref By API String.vi"("Error In (no error)"=w288, "Target Module"=w285) -> ("error out"=w291:errorcluster, "CSM VI Ref"=w292:refnum<vi>)  [unwired: 8 in]
        n106 = control-ref of="LB-Subpnl"() -> (w293:refnum<vi>)
        n107 = invoke class="SubPnl" method="Insert VI"(reference=w293, error in=w291, "VI Ref"=w292) -> (error out=w290:errorcluster)  [unwired: 1 in, 3 out]
      }
      frame "UI: Insert Log Table Window" {
        n108 = call <userlib>:"CSM - Check If Module Exists.vi"("CSM Name"="Log Table Window") -> ("Error out"=w325:errorcluster, "Exist?"=w327:bool, "CSM Name(dup)"=w324:string)  [unwired: 8 in]
        n109 = case shown="False" w327 {
          tunnel: [w339 w358] -> w326
          tunnel: w325 -> [w340 w358]
          tunnel: w324 -> [w338 w357]
          tunnel: [w338 w357] -> w323
          frame False {
            n110 = vi-ref "CSM Log Table Window.vi"() -> (w341:refnum<vi>)
            n111 = property class="VI (strict)"(reference=w341, error in=w340) -> (reference out=w345:refnum<vi>, error out=w344:errorcluster, "Path"=w343:path)
            n112 = Open VI Reference(type specifier VI Refnum (for type only)=w345, vi path=w343, options=128, error in (no error)=w344) -> (vi reference=w337:refnum<vi>, error out=w342:errorcluster)  [unwired: 2 in]
            n113 = disable-structure shown="Disabled" {
              disable-tunnel: w342 -> [w354 w356]
              disable-tunnel: w337 -> [w352 w355]
              disable-tunnel: [w351 w356] -> w336
              disable-tunnel: [w349 w355] -> w335
              frame Disabled {
                n114 = invoke class="VI (strict)" method="FP.Open"(reference=w352, error in=w354, "State"=T3."Hidden") -> (reference out=w349:refnum<vi>, error out=w353:errorcluster)  [unwired: 2 in, 3 out]
                n115 = call <userlib>:"MGI Clear Error.vi"("Error In"=w353) -> ("Error Out"=w351:errorcluster)  [unwired: 6 in]
              }
              frame Enabled {
              }
            }
            n116 = call-by-ref "Start Asynchronous Call"(reference=w335, error in=w336, "Name(\"\" to use uuid)"=w338) -> (reference out=w347:refnum<vi>, error out=w346:errorcluster)  [unwired: 11 in]
            n117 = Close Reference(reference=w347, error in (no error)=w346) -> (error out=w339:errorcluster)
          }
          frame True {
          }
        }
        n118 = call <userlib>:"CSM - Query CSM VI Ref By API String.vi"("Error In (no error)"=w326, "Target Module"=w323) -> ("error out"=w329:errorcluster, "CSM VI Ref"=w330:refnum<vi>)  [unwired: 8 in]
        n119 = control-ref of="Sub Panel"() -> (w322:refnum<vi>)
        n120 = invoke class="SubPnl" method="Insert VI"(reference=w322, error in=w329, "VI Ref"=w330) -> (error out=w328:errorcluster)  [unwired: 1 in, 3 out]
      }
      frame "---------- Macro ----------" {
        n121 = call <vilib>:"Add State(s) to Queue__JKI_lib_State_Machine.vi"("State(s) in (\"\")"=w362) -> ("States Out"=w361:string)  [unwired: 14 in]
      }
      frame "Macro: Initialize" {
        w364 = "Data: Initialize\nInitialize Core Data\nEvents: Register\nUI: Initialize\nUI: Insert Log Table Window\nUI: Insert Intensity Graph Window\nUI: Front Panel State >> Open"  # Data: Initialize Initialize Core Data Events: Register UI: Initialize UI: Insert Log Table Window UI: Insert Intensity Graph Window UI: Front Panel State >> Open
        n122 = call <vilib>:"Add State(s) to Queue__JKI_lib_State_Machine.vi"("State(s) in Front (\"\")"=w364, "State(s) in (\"\")"=w367) -> ("States Out"=w366:string)  [unwired: 13 in]
      }
      frame "Macro: Exit" {
        n123 = Unbundle By Name(w379) -> ("Core.Close Panel on Exit?"=w378:bool)
        n124 = call <userlib>:"CSM - List Modules.vi"() -> ("Module Names"=w371:string[])  [unwired: 10 in, 1 out]
        n125 = call "Filter 1D Array_nevstop.vim"("items to filter"=w370, "array"=w371) -> ("filtered array"=w369:string[])  [unwired: 4 in, 1 out]
        n126 = call <userlib>:"CSM - Build Exit Messages of CSMs.vi"("CSMs"=w369) -> ("States"=w368:string)  [unwired: 14 in]
        n127 = Select(t="UI: Front Panel State >> Close", s=w378, f="") -> (s? t:f=w375:string)
        n128 = call <vilib>:"Add State(s) to Queue__JKI_lib_State_Machine.vi"("State(s) in Front (\"\")"=w368, "State(s) in (\"\")"=w375, "State(s) at Back (\"\")"="Data: Cleanup\nEvents: Unregister\nExit") -> ("States Out"=w373:string)  [unwired: 12 in]
        n129 = call <vilib>:"Add State(s) to Queue__JKI_lib_State_Machine.vi"("State(s) in Front (\"\")"=w373, "State(s) in (\"\")"=w381) -> ("States Out"=w380:string)  [unwired: 13 in]
      }
      frame "---------- API ----------" {
      }
      frame "API: Load CSMLog File" {
        w386 = "file loader"  # Name("" to use uuid)
        n130 = vi-ref "CSM - File Loader.vi"() -> (w397:refnum<vi>)
        n131 = property class="VI (strict)"(reference=w397) -> (reference out=w393:refnum<vi>, error out=w395:errorcluster, "Path"=w396:path)  [unwired: 1 in]
        n132 = Open VI Reference(type specifier VI Refnum (for type only)=w393, vi path=w396, options=128, error in (no error)=w395) -> (vi reference=w394:refnum<vi>, error out=w398:errorcluster)  [unwired: 2 in]
        n133 = call-by-ref "Start Asynchronous Call"(reference=w394, error in=w398, "Name(\"\" to use uuid)"=w386) -> (reference out=w391:refnum<vi>, error out=w392:errorcluster)  [unwired: 11 in]
        n134 = Close Reference(reference=w391, error in (no error)=w392) -> (error out=w385:errorcluster)
        n135 = call-poly <userlib>:"Build Message with Arguments++.vi"("States with Replace Token"="CSMLOG Snippet@<target> >> API: Snippet Handler@Process -><register>\nAPI: Clear -@ FileMemory\nParsed Log Snippet@Process >> Handler: Record Snippets@FileMemory -><register>\nAPI: Load CSMLOG File >> <param> ->| <target>" ("State(s) in Front (\"\")"), "<param>"=w387, "<target>"=w386) -> ("States"=w389:string)  [unwired: 12 in]
        n136 = call <vilib>:"Add State(s) to Queue__JKI_lib_State_Machine.vi"("State(s) in Front (\"\")"=w389, "State(s) in (\"\")"=w399) -> ("States Out"=w400:string)  [unwired: 13 in]
      }
      frame "Handler: File Size" {
      }
      frame "---------- Action ----------" {
        n137 = call <vilib>:"Add State(s) to Queue__JKI_lib_State_Machine.vi"("State(s) in (\"\")"=w409) -> ("States Out"=w408:string)  [unwired: 14 in]
      }
      frame "Action: action1" {
        n138 = call <vilib>:"Add State(s) to Queue__JKI_lib_State_Machine.vi"("State(s) in (\"\")"=w413) -> ("States Out"=w412:string)  [unwired: 14 in]
      }
      frame "Action: action2" {
        n139 = call <vilib>:"Add State(s) to Queue__JKI_lib_State_Machine.vi"("State(s) in (\"\")"=w417) -> ("States Out"=w416:string)  [unwired: 14 in]
      }
    }
  }
  n140 = call "CSM - Process Module.vi"("Name(\"\" to use uuid)"=w4) -> ()  [unwired: 11 in]
  n141 = call "CSM - Process Module.vi"("Name(\"\" to use uuid)"=w4) -> ()  [unwired: 11 in]
  n142 = call "CSM - Process Module.vi"("Name(\"\" to use uuid)"=w4) -> ()  [unwired: 11 in]
  n143 = call "CSM - Process Module.vi"("Name(\"\" to use uuid)"=w4) -> ()  [unwired: 11 in]
  n144 = call "CSM - LogMem.vi"("Name(\"\" to use uuid)"="FileMemory" ("Name(\"\" to use uuid)")) -> ()  [unwired: 11 in]
  n145 = disable-structure shown="Disabled" {
    frame Disabled {
      n146 = call <userlib>:"Trim Both Whitespace.vi"("string"="") -> ("trimmed string"=→"data":string)  [unwired: 1 in]
      n147 = Scan From String(format string="%<%Y/%m/%d %H:%M:%S%3u>T", default 1=timestamp(0 s since 1904-01-01)) -> (output 1=w420:timestamp)  [unwired: 3 in, 3 out]
      n148 = Format Into String(format string="%<%Y/%m/%d %H:%M:%S>T", w420) -> ()  [unwired: 2 in, 2 out]
    }
    frame Enabled {
    }
  }
  n149 = disable-structure shown="Disabled" {
    frame Disabled {
      n150 = Get Variant Attribute() -> (names=w437:string[], values=w438:variant[])  [unwired: 4 in, 2 out]
      n151 = Get Variant Attribute() -> (names=w433:string[], values=w434:variant[])  [unwired: 4 in, 2 out]
      n152 = Variant To Data(type=i64[] [] ("offset (in bytes) (0)"), Variant=w434) -> (data=w432:i64[])  [unwired: 1 in, 1 out]
      n153 = Variant To Data(type=i64[] [] ("offset (in bytes) (0)"), Variant=w438) -> (data=w439:i64[])  [unwired: 1 in, 1 out]
      n154 = for {
        tunnel: w433 -> [w451] mode=indexing
        tunnel: w432 -> [w446] mode=indexing
        tunnel: [w444] -> w431 mode=indexing if=w440
        n155 = call <userlib>:"String to 1D Array_csm.vi"("delimiter (Tab)"="|", "string"=w451) -> ("Array of Strings"=w449:string[])  [unwired: 9 in]
        n156 = for {
          tunnel: w449 -> [w453] mode=indexing
          tunnel: [w452] -> w448 mode=indexing
          n157 = call <userlib>:"Trim Both Whitespace.vi"("string"=w453) -> ("trimmed string"=w452:string)  [unwired: 1 in]
        }
        n158 = Format Into String(w446) -> (resulting string=w445:string)  [unwired: 3 in, 1 out]
        n159 = call <userlib>:"1D Array to String_csm.vi"("delimiter (Tab)"="/", "Array of Strings"=w448) -> ("delimited string"=w443:string)  [unwired: 9 in]
        n160 = Build Array(w443, w445) -> (w444:string[])
        n161 = Match Pattern(string=w443, regular expression="(Complete)$") -> (offset past match=w441:i32)  [unwired: 1 in, 3 out]
        n162 = Less Than 0?(x=w441) -> (x < 0?=w440:bool)
      }
      n163 = for {
        tunnel: w437 -> [w457] mode=indexing
        tunnel: w439 -> [w455] mode=indexing
        tunnel: [w454] -> w427 mode=indexing
        n164 = Scan From String(format string="%<%Y/%m/%d %H:%M:%S>T", input string=w457) -> (output 1=w456:timestamp)  [unwired: 3 in, 3 out]
        n165 = Bundle(w456, "offset (in bytes) (0)"=w455) -> (w454:cluster{timestamp, "offset (in bytes) (0)":i64})  [unwired: 1 in]
      }
      n166 = control-ref of="Tree"() -> (w429:refnum<vi>)
      n167 = call <userlib>:"MGI Populate Tree with Delimited Strings.vi"("Delimiter"="/" ("delimiter (Tab)"), "Items (Delimited)"=w431, "Tree Control"=w429) -> ()  [unwired: 6 in, 3 out]
      n168 = call "CSM - Convert MassData to Argument.vim"("DBL"=w427) -> ("error out"=w425:errorcluster, "MassData Argument"=w426:string)  [unwired: 7 in]
      n169 = call <userlib>:"CSM - Post Message.vi"("Error In (no error)"=w425, "Target Module"="CSM", "Arguments (\"\")"=w426, "State"="API: Add Points") -> ()  [unwired: 7 in, 1 out]
    }
    frame Enabled {
    }
  }
